vi "Read Control Label.vi"(8 "error in (no error)":errorcluster, 11 "ControlDropMsg In":refnum<class "ControlDropMsg.lvclass">) -> (0 "error out":errorcluster, 2 "Control Label":string, 3 "ControlDropMsg Out":refnum<class "ControlDropMsg.lvclass">)   [LabVIEW 2020, in "ActorEvents.lvlib" / "ControlDropMsg.lvclass"]
uses:
  <vilib>/gpm_packages/@cs/mva-viewable/Source/ActorEvents/IEventAggregator Messages/ControlDropMsg/ControlDropMsg.lvclass
  <vilib>/gpm_packages/@cs/mva-viewable/Source/ActorEvents/IEventAggregator Messages/ControlDropMsg/ControlDropMsg.lvclass/ControlDropMsg.ctl
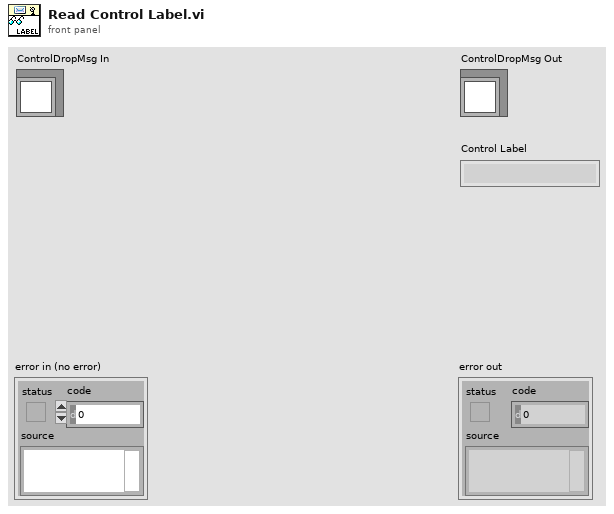
[diagram p1: front panel]
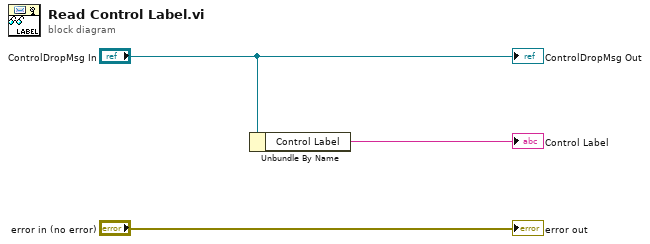
[diagram p0: block diagram]
diagram:
  n1 = Unbundle By Name("ControlDropMsg In") -> ("Control Label"=→"Control Label":string)
  "error out" <- "error in (no error)"
  "ControlDropMsg Out" <- "ControlDropMsg In"
